vi "Bitmap File Writer.vi"   [LabVIEW 2010]
uses:
  Instance           1 26Saved   Bitmap File Writer .vi
types:
  T1 = enum16{"open", "replace", "create", "open or create", "replace or create", "replace or create with confirmation"}
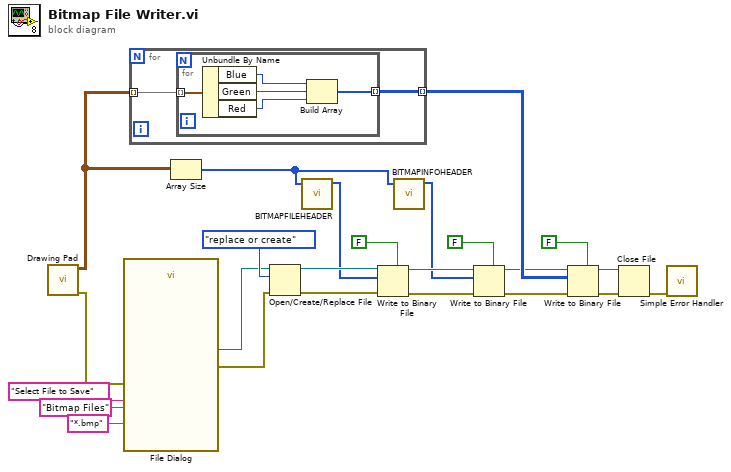
[diagram p0: block diagram]
diagram:
  n1 = call "Drawing Pad.vi"() -> ("error out"=w4:errorcluster, "Image Data"=w14:cluster{"Red":u8, "Green":u8, "Blue":u8}[][])  [unwired: 10 in]
  n2 = call "File Dialog"("prompt"="Select File to Save", "error in"=w4, "pattern (all files)"="*.bmp", "pattern label"="Bitmap Files") -> ("selected path"=w6:path, "error out"=w5:errorcluster)  [unwired: 8 in, 2 out]
  n3 = for {
    tunnel: w14 -> [w26] mode=indexing
    tunnel: [w25] -> w12 mode=indexing
    n4 = for {
      tunnel: w26 -> [w31] mode=indexing
      tunnel: [w27] -> w25 mode=indexing
      n5 = Unbundle By Name(w31) -> ("Blue"=w29:u8, "Green"=w30:u8, "Red"=w28:u8)
      n6 = Build Array(w29, w30, w28) -> (w27:u8[])
    }
  }
  n7 = Array Size(array=w14) -> (size(s)=w17:i32[])
  n8 = Open/Create/Replace File(file path (use dialog)=w6, error in=w5, operation (0:open)=T1."replace or create") -> (refnum out=w21:refnum<file>, error out=w20:errorcluster)  [unwired: 3 in, 1 out]
  n9 = call "BITMAPFILEHEADER.vi"("Image Dimensions"=w17) -> ("BITMAPFILEHEADER"=w16:u8[])  [unwired: 10 in]
  n10 = Write to Binary File(file (use dialog)=w21, data=w16, error in=w20, 5:FALSE ("prepend array or string size? (T)")) -> (refnum out=w19:refnum<file>, error out=w18:errorcluster)  [unwired: 2 in, 1 out]
  n11 = call "BITMAPINFOHEADER.vi"("Image Dimensions"=w17) -> ("BITMAPFILEHEADER"=w15:u8[])  [unwired: 10 in]
  n12 = Write to Binary File(file (use dialog)=w19, data=w15, error in=w18, 5:FALSE ("prepend array or string size? (T)")) -> (refnum out=w11:refnum<file>, error out=w10:errorcluster)  [unwired: 2 in, 1 out]
  n13 = Write to Binary File(file (use dialog)=w11, data=w12, error in=w10, 5:FALSE ("prepend array or string size? (T)")) -> (refnum out=w8:refnum<file>, error out=w9:errorcluster)  [unwired: 2 in, 1 out]
  n14 = Close File(refnum=w8, error in=w9) -> (error out=w7:errorcluster)  [unwired: 1 out]
  n15 = call <vilib>:"Simple Error Handler.vi"("error in (no error)"=w7) -> ()  [unwired: 4 in, 5 out]
